vi "Data.vi"(11 "Merge Error Msg in":refnum<class "Merge Error Msg.lvclass">) -> (2 "Error":errorcluster)   [LabVIEW 2021, in "Merge Error.lvlib" / "Merge Error Msg.lvclass"]
uses:
  Merge Error Msg.lvclass
  Merge Error Msg.lvclass/Merge Error Msg.ctl
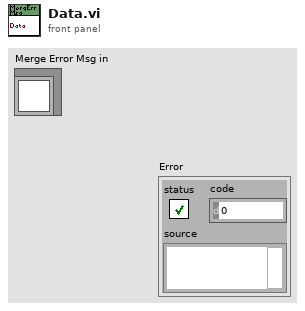
[diagram p1: front panel]
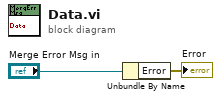
[diagram p0: block diagram]
diagram:
  n1 = Unbundle By Name("Merge Error Msg in") -> ("Error"=→"Error":errorcluster)
